vi "FPGA Main.vi"   [LabVIEW 2020]
uses:
  <vilib>/rvi/Emulation/niFpgaGetClockAttributes.vi
  <vilib>/rvi/Emulation/niFpgaSctlEmulationGetInTimedLoop.vi
  <vilib>/rvi/Emulation/niFpgaEmulationReportErrorSimple.vi
  <vilib>/rvi/eio/common/nirviEmuTemplateMethod_errors.vi
  <vilib>/rvi/Emulation/niFpgaCriticalErrorInLSC.vi
  <vilib>/eio/EIONode/EIONode.xnode
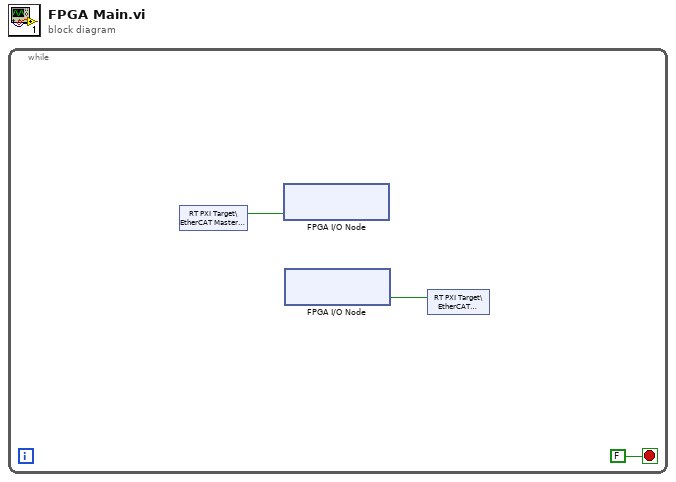
[diagram p0: block diagram]
diagram:
  n1 = while {
    stop <- FALSE stop-if-true
    n2 = shared-variable "RT PXI Target\\EtherCAT Master\\Device\\User-Defined Variables\\DO0"() -> (w1:bool)  [unwired: 1 in, 1 out]
    n3 = xnode "FPGA I/O Node"("Mod8/DIO0"=w1) -> ()  [unwired: 1 in, 1 out]
    n4 = xnode "FPGA I/O Node"() -> ("Mod8/DIO4"=w2:bool)  [unwired: 1 in, 1 out]
    n5 = shared-variable "RT PXI Target\\EtherCAT Master\\Device\\User-Defined Variables\\DI4"(w2) -> ()  [unwired: 1 in, 1 out]
  }
